vi "ME and SD.vi"(0 "Array":dbl[][](array[numeric]), 1 "Sorted Probabilities":cluster{dbl, dbl, i32}[](array[cluster])) -> (3 "SD":dbl[](array[numeric]), 4 "ME":dbl[](array[numeric]))   [LabVIEW 2018]
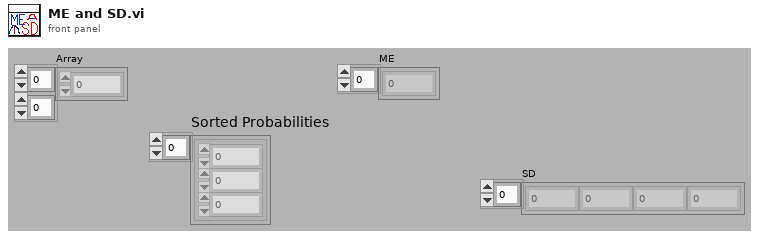
[diagram p1: front panel]
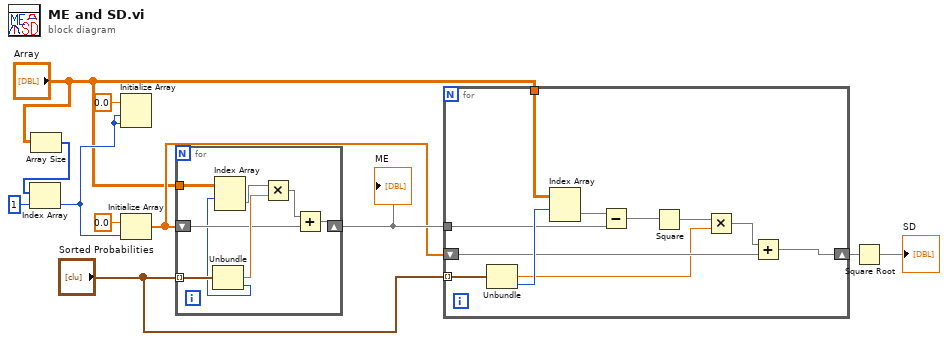
[diagram p0: block diagram]
diagram:
  n1 = Array Size(array="Array") -> (size(s)=w10:i32[])
  n2 = Index Array(array=w10, index=1) -> (element=w2:i32)
  n3 = Initialize Array(0.0 ("element"), w2, w2) -> ()  [unwired: 1 out]
  n4 = Initialize Array(0.0 ("element"), w2) -> (w6:dbl[])
  n5 = for {
    tunnel: "Array" -> [w17]
    tunnel: "Sorted Probabilities" -> [w19] mode=indexing
    shift-right: [w16] -> w7
    shift-left: w6 -> [w15]
    n6 = Unbundle(w19) -> (w18:dbl, w13:i32)  [unwired: 1 out]
    n7 = Index Array(array=w17, index (row)=w13) -> (element=w14:dbl[])  [unwired: 1 in]
    n8 = Multiply(x=w14, y=w18) -> (x*y=w12:dbl[])
    n9 = Add(x=w12, y=w15) -> (x+y=w16:dbl[])
  }
  "ME" <- w7
  n10 = for {
    tunnel: "Array" -> [w29]
    tunnel: "Sorted Probabilities" -> [w30] mode=indexing
    tunnel: w7 -> [w27]
    shift-right: [w23] -> w5
    shift-left: w6 -> [w24]
    n11 = Unbundle(w30) -> (w21:dbl, w28:i32)  [unwired: 1 out]
    n12 = Index Array(array=w29, index (row)=w28) -> (element=w22:dbl[])  [unwired: 1 in]
    n13 = Subtract(x=w22, y=w27) -> (x-y=w20:dbl[])
    n14 = Square(x=w20) -> (x^2=w26:dbl[])
    n15 = Multiply(x=w26, y=w21) -> (x*y=w25:dbl[])
    n16 = Add(x=w25, y=w24) -> (x+y=w23:dbl[])
  }
  n17 = Square Root(x=w5) -> (sqrt(x)=→"SD":dbl[])
